vi "udpBroadcast.vi"(10 "remote port":u16, 11 "data in":string) -> ()   [LabVIEW 2017]
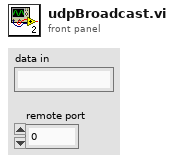
[diagram p1: front panel]
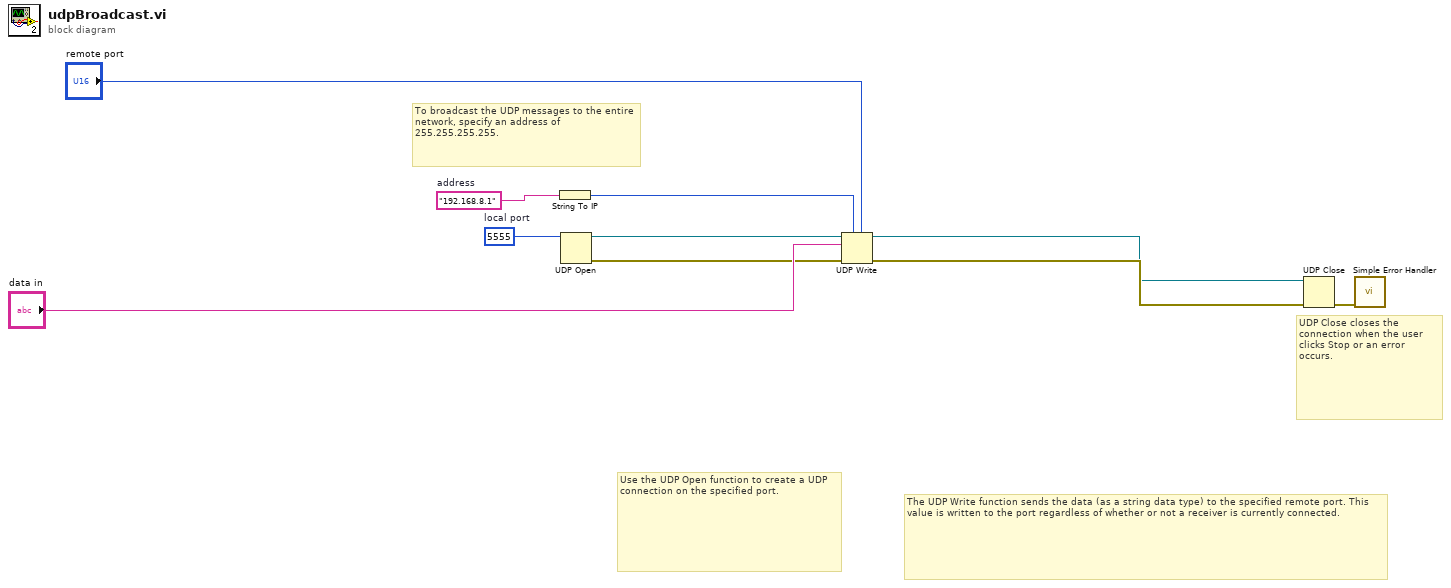
[diagram p0: block diagram]
diagram:
  w8 = u16 5555  # local port
  w3 = "192.168.8.1"  # address
  # "To broadcast the UDP messages to the entire network, specify an address of 255.255.255.255."
  # "UDP Close closes the connection when the user clicks Stop or an error occurs."
  # "The UDP Write function sends the data (as a string data type) to the specified remote port. This value is written to the port regardless of whether or not a receiver is currently connected."
  # "Use the UDP Open function to create a UDP connection on the specified port."
  n1 = String To IP(1:w3) -> (0:w5:u32)
  n2 = UDP Open(11:w8) -> (port=w6:refnum<k16>, 0:w7:errorcluster)  [unwired: 4 in, 1 out]
  n3 = UDP Write(address=w5, port or service name="remote port", connection ID=w6, data in="data in", 8:w7) -> (error out=w2:errorcluster, 3:w1:refnum<k16>)  [unwired: 1 in]
  n4 = UDP Close(connection ID=w1, 8:w2) -> (error out=w4:errorcluster)  [unwired: 1 out]
  n5 = call <vilib>:"Simple Error Handler.vi"("error in (no error)"=w4) -> ()  [unwired: 4 in, 5 out]
